vi "user interface.vi"(11 "Serial port assistant view":refnum<class "Serial port assistant view.lvclass">) -> ()   [LabVIEW 2022 SP3, in "Serial port assistant view.lvlib" / "Serial port assistant view.lvclass"]
uses:
  Serial port assistant view.lvclass
  Serial port assistant view.lvclass/Serial port assistant view.ctl
panel:
  in  "open?":bool
  in  "发送间隔":u32
  in  "定时发送？":bool
  in  "HEX？":bool
  in  "清空显示":bool
  in  "HEX显示？":bool
  in  "发送":bool
  in  "发送数据":string
  in  "停止位":string(combo)="1"
  in  "校验位":string(combo)="none"
  in  "数据位":string(combo)="8"
  in  "波特率":string(combo)="9600"
  in  "串口号":string(combo)
  in  "打开串口":bool
  out "实时显示":string
  # "串口设置"
  # "串口设置"
  # "设置"
  # "实时显示"
  # "发送"
  # "发送间隔(ms)"
  # "定时发送"
  # "HEX"
  # "HEX显示"
  # "停止位："
  # "校验位："
  # "数据位："
  # "波特率："
  # "串口号："
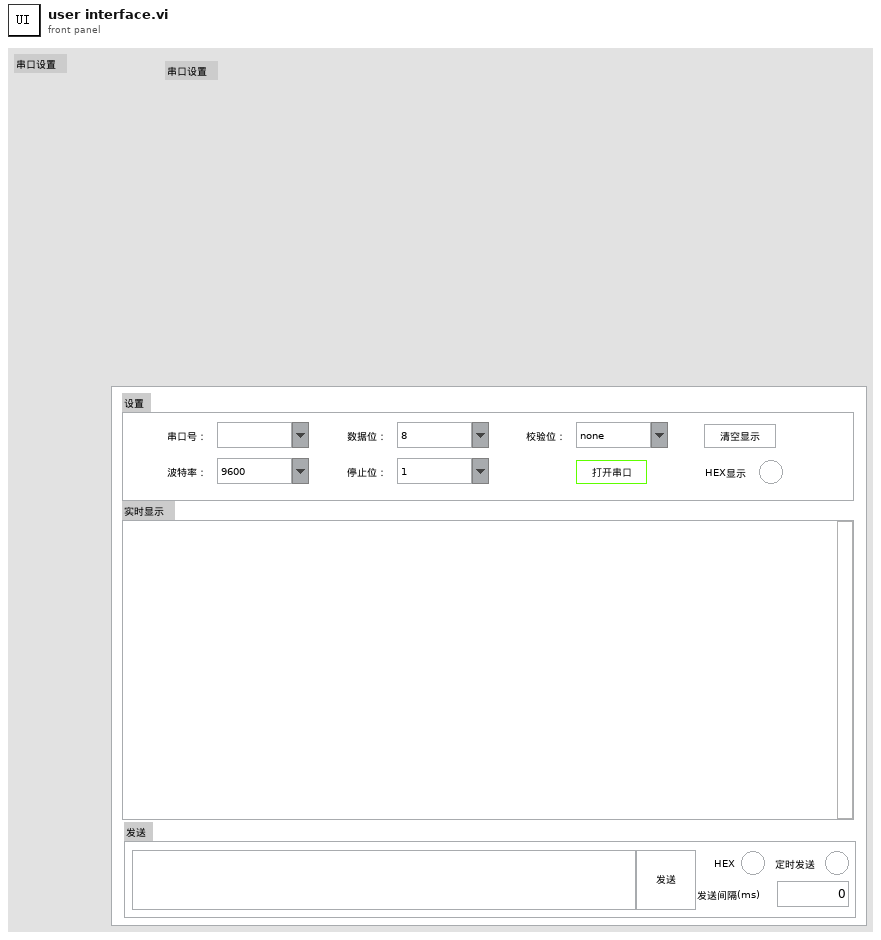
[diagram p1: front panel]
types:
  T1 = cluster{"request":string, "serial port":string, "baud rate":u32, "data bits":u16, "stop bits":u16, "parity":u16}
  T2 = cluster{"request":string, "data to be sent":string}
  T3 = enum8{"Enabled", "Disabled", "Disabled and Grayed Out"}
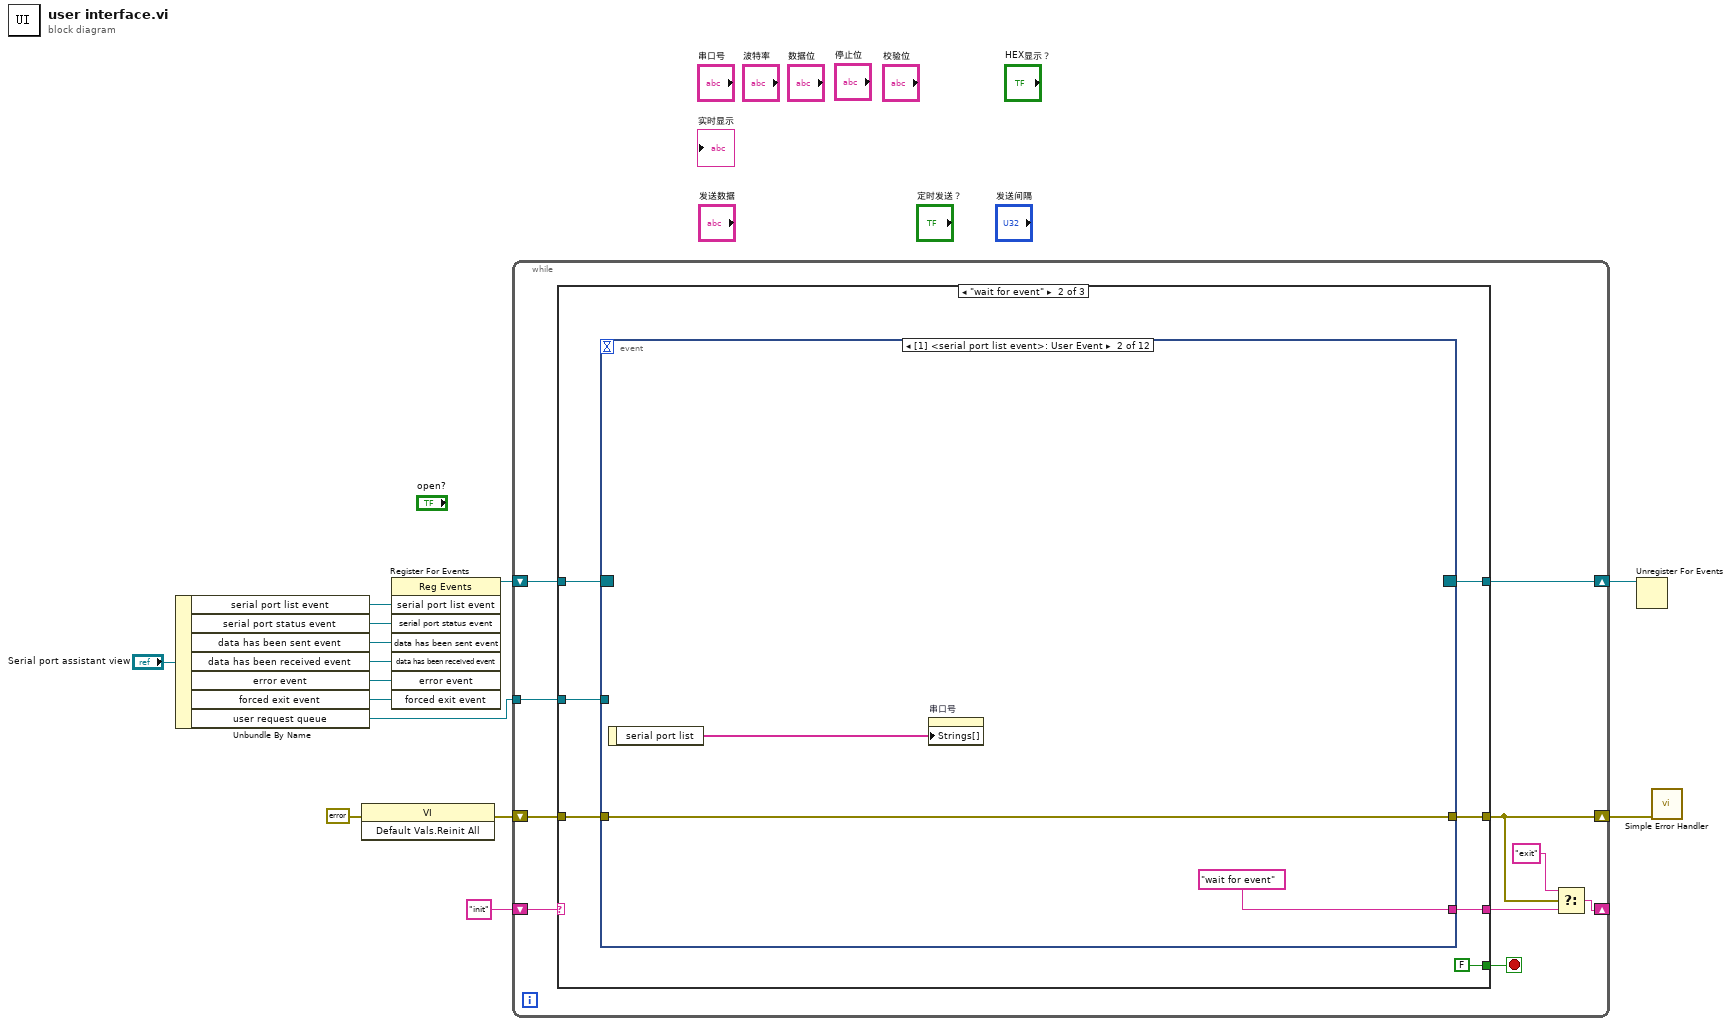
[diagram p0: block diagram]
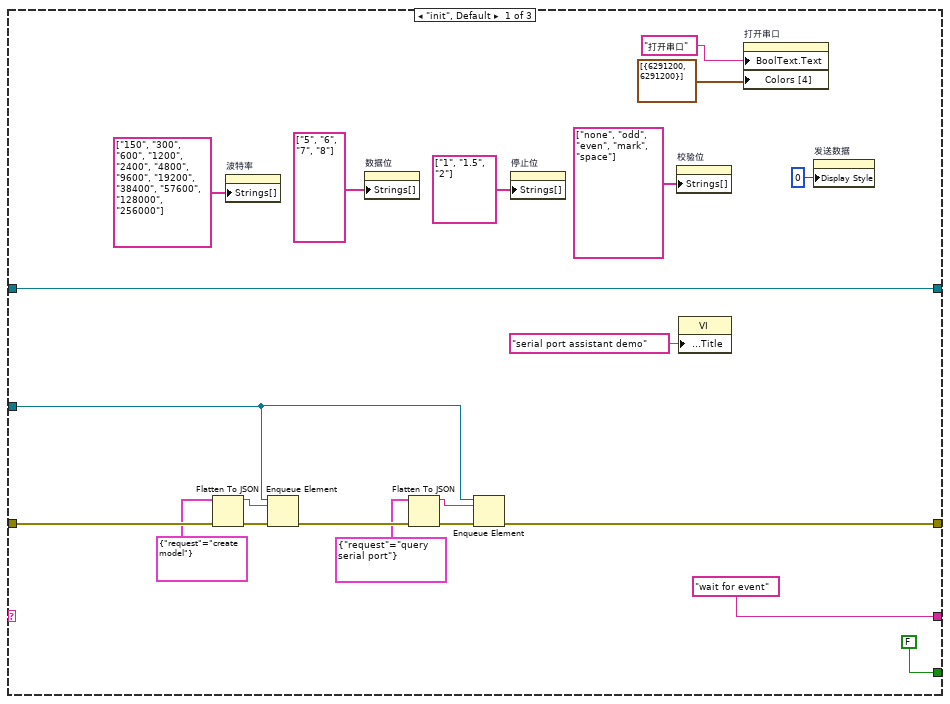
[diagram p2: hidden frame]
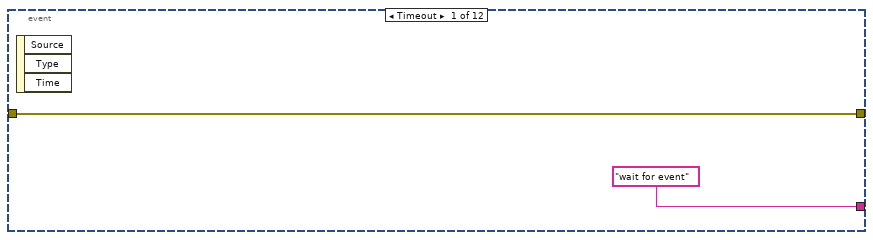
[diagram p3: hidden frame]
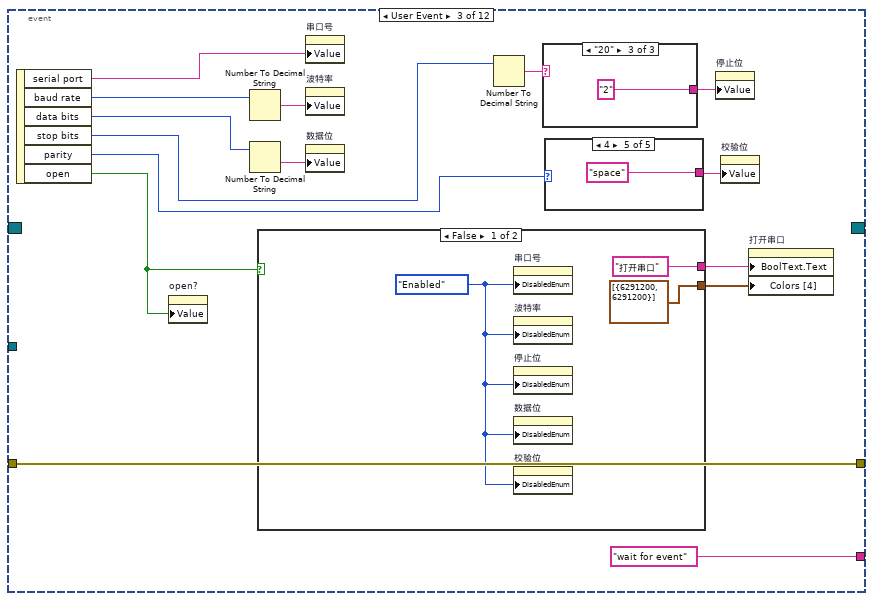
[diagram p4: hidden frame]
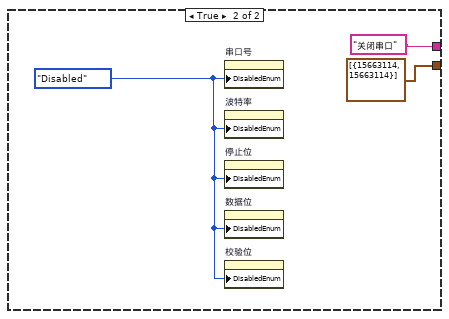
[diagram p5: hidden frame]
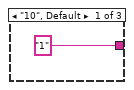
[diagram p6: hidden frame]
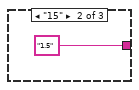
[diagram p7: hidden frame]
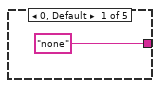
[diagram p8: hidden frame]
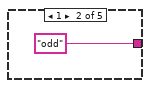
[diagram p9: hidden frame]
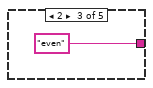
[diagram p10: hidden frame]
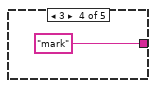
[diagram p11: hidden frame]
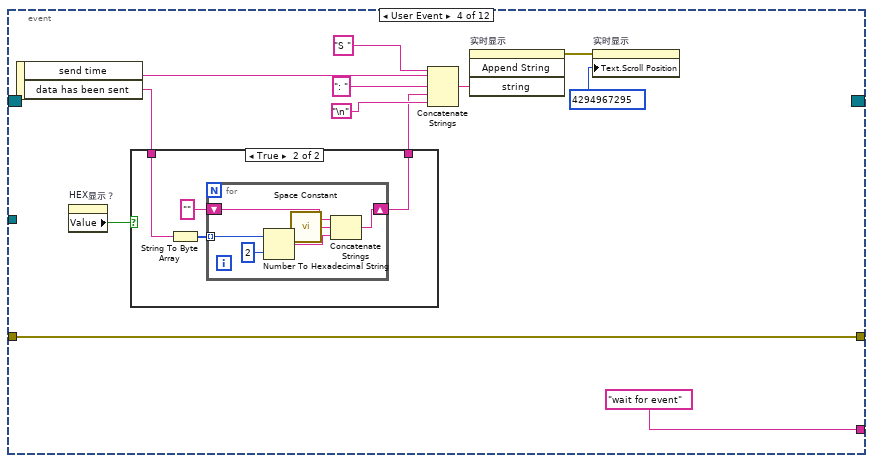
[diagram p12: hidden frame]
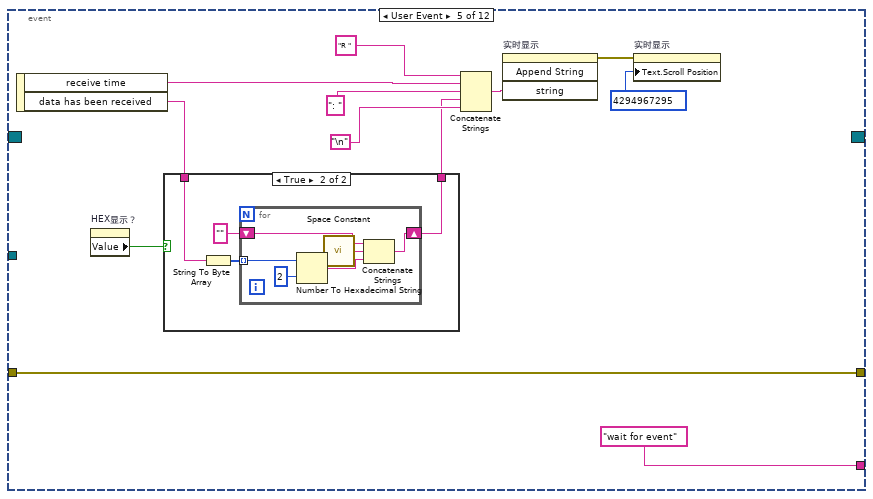
[diagram p14: hidden frame]
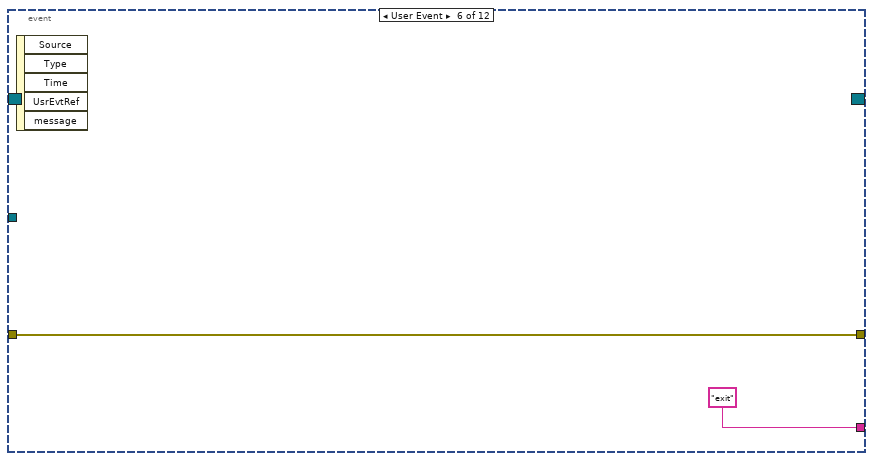
[diagram p16: hidden frame]
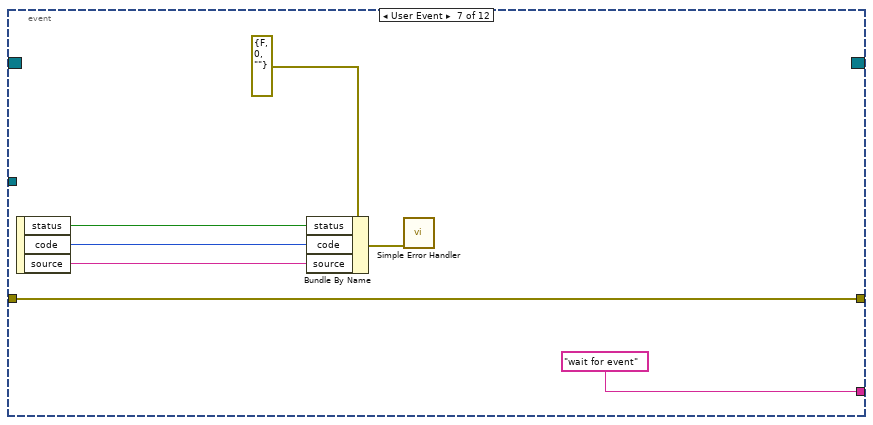
[diagram p17: hidden frame]
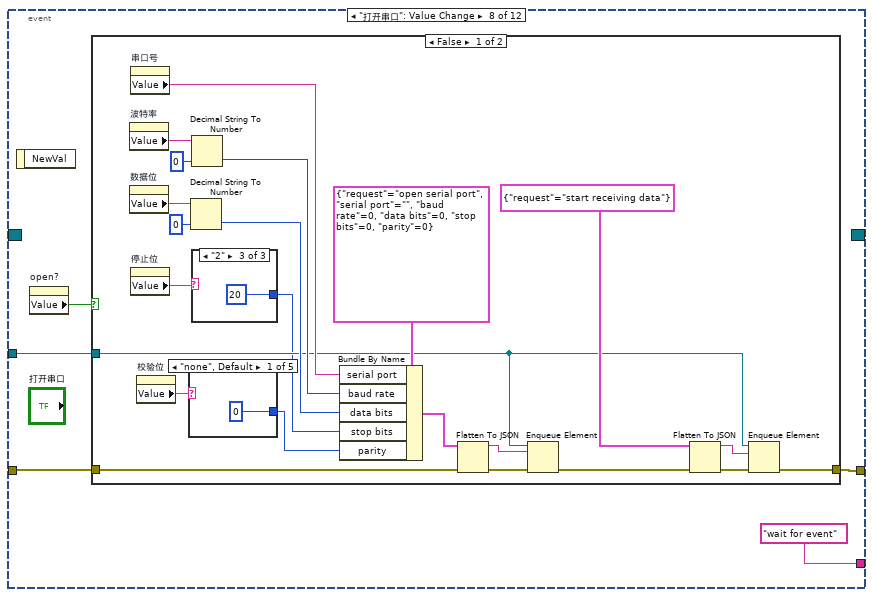
[diagram p18: hidden frame]
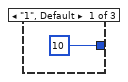
[diagram p19: hidden frame]
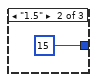
[diagram p20: hidden frame]
diagram:
  n1 = Unbundle By Name("Serial port assistant view") -> ("serial port list event"=w13:refnum<user-event>, "serial port status event"=w12:refnum<user-event>, "data has been sent event"=w11:refnum<user-event>, "data has been received event"=w10:refnum<user-event>, "error event"=w7:refnum<user-event>, "forced exit event"=w2:refnum<user-event>, "user request queue"=w1:refnum<queue>)
  n2 = invoke class="VI" method="Default Vals.Reinit All"(error in=errorcluster {"status"=FALSE, "code"=0, "source"=""} ("error in (no error)")) -> (error out=w5:errorcluster)  [unwired: 2 in, 2 out]
  n3 = register-events(w13, w12, w11, w10, w7, w2) -> (reference out=w9:refnum<event-registration>)  [unwired: 2 in, 1 out]
  n4 = while {
    shift-right: [w19] -> w8
    shift-left: w5 -> [w23]
    tunnel: w1 -> [w22]
    shift-right: [w16] -> _
    shift-left: "init" -> [w21]
    shift-right: [w20] -> w3
    shift-left: w9 -> [w24]
    stop <- w18 stop-if-true
    n5 = case shown="\"wait for event\"" w21 {
      tunnel: w24 -> [w45 w52 w266]
      tunnel: [w45 w51 w266] -> w20
      tunnel: w23 -> [w38 w50 w259]
      tunnel: w22 -> [w37 w49 w261]
      tunnel: [w36 w48 w258] -> w19
      tunnel: [FALSE FALSE TRUE ("Discard?")] -> w18
      tunnel: ["wait for event" w47 "exit"] -> w17
      frame "init", Default {
        n6 = Flatten To JSON(anything=cluster{"request":string} {"request"="create model"}, error in (no error)=w38) -> (JSON string=w43:string, 11:w40:errorcluster)  [unwired: 1 in]
        n7 = property on="波特率" class="CmbBox"("Strings[]"=string[] ["150", "300", "600", "1200", "2400", "4800", "9600", "19200", "38400", "57600", "128000", "256000"] ("Strings [] 5")) -> ()  [unwired: 2 in, 2 out]
        n8 = Enqueue Element(queue=w37, element=w43, error in (no error)=w40) -> (error out=w41:errorcluster)  [unwired: 1 in, 2 out]
        n9 = property on="数据位" class="CmbBox"("Strings[]"=string[] ["5", "6", "7", "8"] ("Strings [] 5")) -> ()  [unwired: 2 in, 2 out]
        n10 = Flatten To JSON(anything=cluster{"request":string} {"request"="query serial port"}, error in (no error)=w41) -> (JSON string=w44:string, 11:w42:errorcluster)  [unwired: 1 in]
        n11 = Enqueue Element(queue=w37, element=w44, error in (no error)=w42) -> (error out=w36:errorcluster)  [unwired: 1 in, 2 out]
        n12 = property on="停止位" class="CmbBox"("Strings[]"=string[] ["1", "1.5", "2"] ("Strings [] 5")) -> ()  [unwired: 2 in, 2 out]
        n13 = property on="校验位" class="CmbBox"("Strings[]"=string[] ["none", "odd", "even", "mark", "space"] ("Strings [] 5")) -> ()  [unwired: 2 in, 2 out]
        n14 = property class="VI"("Front Panel.Title"="serial port assistant demo" ("Front Panel Window:Title")) -> ()  [unwired: 2 in, 2 out]
        n15 = property on="打开串口" class="Bool"("BoolText.Text"="打开串口", "Colors [4]"=cluster{u32, u32}[] [{6291200, 6291200}]) -> ()  [unwired: 2 in, 2 out]
        n16 = property on="发送数据" class="Str"("Display Style"=u32 0) -> ()  [unwired: 2 in, 2 out]
      }
      frame "wait for event" {
        n17 = event shown="[1] <serial port list event>: User Event" {
          selector: w52 -> [_ _ _ _ _ _ _ _ _ _ _ _]
          dyn-events: [_ _ _ _ _ _ _ _ _ _ _ _] -> w51
          timeout: _ -> [_ _ _ _ _ _ _ _ _ _ _ _]
          tunnel: w50 -> [w54 w56 w67 w96 w119 w133 w141 w145 w188 w195 w215 w222]
          tunnel: [w54 w56 w67 w96 w119 w133 w141 w144 w188 w194 w215 w224] -> w48
          tunnel: w49 -> [_ _ _ _ _ _ _ w143 _ w193 _ w223]
          tunnel: ["wait for event" "wait for event" "wait for event" "wait for event" "wait for event" "exit" "wait for event" "wait for event" "wait for event" "wait for event" "wait for event" w220] -> w47
          event Timeout {
            n18 = event-data() -> ()  [unwired: 1 in, 3 out]
          }
          event User Event {
            n19 = event-data() -> ("serial port list"=w57:string[])  [unwired: 1 in]
            n20 = property on="串口号" class="CmbBox"("Strings[]"=w57) -> ()  [unwired: 2 in, 2 out]
          }
          event User Event {
            n21 = event-data() -> ("serial port"=w72:string, "baud rate"=w71:u32, "data bits"=w68:u16, "stop bits"=w58:u16, "parity"=w65:u16, "open"=w61:bool)  [unwired: 1 in]
            n22 = property on="open?" class="Bool (strict)"("Value"=w61) -> ()  [unwired: 2 in, 2 out]
            n23 = Number To Decimal String(number=w71) -> (decimal integer string=w70:string)  [unwired: 1 in]
            n24 = Number To Decimal String(number=w68) -> (decimal integer string=w69:string)  [unwired: 1 in]
            n25 = case shown="False" w61 {
              tunnel: ["打开串口" "关闭串口"] -> w60
              tunnel: [cluster{u32, u32}[] [{6291200, 6291200}] ("Colors [4]") cluster{u32, u32}[] [{15663114, 15663114}] ("Colors [4]")] -> w59
              frame False {
                w73 = T3."Enabled" ("Disabled")
                n26 = property on="串口号" class="CmbBox"("DisabledEnum"=w73) -> ()  [unwired: 2 in, 2 out]
                n27 = property on="波特率" class="CmbBox"("DisabledEnum"=w73) -> ()  [unwired: 2 in, 2 out]
                n28 = property on="停止位" class="CmbBox"("DisabledEnum"=w73) -> ()  [unwired: 2 in, 2 out]
                n29 = property on="数据位" class="CmbBox"("DisabledEnum"=w73) -> ()  [unwired: 2 in, 2 out]
                n30 = property on="校验位" class="CmbBox"("DisabledEnum"=w73) -> ()  [unwired: 2 in, 2 out]
              }
              frame True {
                w76 = T3."Disabled" ("Disabled")
                n31 = property on="串口号" class="CmbBox"("DisabledEnum"=w76) -> ()  [unwired: 2 in, 2 out]
                n32 = property on="波特率" class="CmbBox"("DisabledEnum"=w76) -> ()  [unwired: 2 in, 2 out]
                n33 = property on="停止位" class="CmbBox"("DisabledEnum"=w76) -> ()  [unwired: 2 in, 2 out]
                n34 = property on="数据位" class="CmbBox"("DisabledEnum"=w76) -> ()  [unwired: 2 in, 2 out]
                n35 = property on="校验位" class="CmbBox"("DisabledEnum"=w76) -> ()  [unwired: 2 in, 2 out]
              }
            }
            n36 = property on="串口号" class="CmbBox"("Value"=w72) -> ()  [unwired: 2 in, 2 out]
            n37 = property on="波特率" class="CmbBox"("Value"=w70) -> ()  [unwired: 2 in, 2 out]
            n38 = property on="数据位" class="CmbBox"("Value"=w69) -> ()  [unwired: 2 in, 2 out]
            n39 = Number To Decimal String(number=w58) -> (decimal integer string=w63:string)  [unwired: 1 in]
            n40 = case shown="\"20\"" w63 {
              tunnel: ["1" "1.5" "2"] -> w62
              frame "10", Default {
              }
              frame "15" {
              }
              frame "20" {
              }
            }
            n41 = case shown="4" w65 {
              tunnel: ["none" "odd" "even" "mark" "space"] -> w64
              frame 0, Default {
              }
              frame 1 {
              }
              frame 2 {
              }
              frame 3 {
              }
              frame 4 {
              }
            }
            n42 = property on="停止位" class="CmbBox"("Value"=w62) -> ()  [unwired: 2 in, 2 out]
            n43 = property on="校验位" class="CmbBox"("Value"=w64) -> ()  [unwired: 2 in, 2 out]
            n44 = property on="打开串口" class="Bool"("BoolText.Text"=w60, "Colors [4]"=w59) -> ()  [unwired: 2 in, 2 out]
          }
          event User Event {
            n45 = event-data() -> ("send time"=w92:string, "data has been sent"=w88:string)  [unwired: 1 in]
            n46 = property on="HEX显示？" class="Bool (strict)"() -> ("Value"=w89:bool)  [unwired: 2 in, 2 out]
            n47 = case shown="True" w89 {
              tunnel: w88 -> [w99 w101]
              tunnel: [w99 w100] -> w87
              frame False {
              }
              frame True {
                n48 = String To Byte Array(string=w101) -> (unsigned byte array=w102:u8[])
                n49 = for {
                  tunnel: w102 -> [w108] mode=indexing
                  shift-right: [w106] -> w100
                  shift-left: "" -> [w107]
                  n50 = Number To Hexadecimal String(1:i16 2 ("width (-)"), 2:w108) -> (0:w105:string)
                  n51 = call <vilib>:"Space Constant.vi"() -> ("String"=w104:string)
                  n52 = Concatenate Strings(w107, w104, w105) -> (w106:string)
                }
              }
            }
            n53 = Concatenate Strings("S " ("string"), w92, ": ", w87, "\n") -> (w94:string)
            n54 = invoke on="实时显示" class="Str" method="Append String"("string"=w94) -> (error out=w98:errorcluster)  [unwired: 3 in, 3 out]
            n55 = property on="实时显示" class="Str"(error in=w98, "Text.Scroll Position"=u32 4294967295) -> ()  [unwired: 1 in, 2 out]
          }
          event User Event {
            n56 = event-data() -> ("receive time"=w114:string, "data has been received"=w111:string)  [unwired: 1 in]
            n57 = property on="HEX显示？" class="Bool (strict)"() -> ("Value"=w112:bool)  [unwired: 2 in, 2 out]
            n58 = case shown="True" w112 {
              tunnel: w111 -> [w122 w124]
              tunnel: [w122 w123] -> w110
              frame False {
              }
              frame True {
                n59 = String To Byte Array(string=w124) -> (unsigned byte array=w125:u8[])
                n60 = for {
                  tunnel: w125 -> [w131] mode=indexing
                  shift-right: [w129] -> w123
                  shift-left: "" -> [w130]
                  n61 = Number To Hexadecimal String(1:i16 2 ("width (-)"), 2:w131) -> (0:w128:string)
                  n62 = call <vilib>:"Space Constant.vi"() -> ("String"=w127:string)
                  n63 = Concatenate Strings(w130, w127, w128) -> (w129:string)
                }
              }
            }
            n64 = Concatenate Strings("R " ("string"), w114, ": ", w110, "\n") -> (w113:string)
            n65 = invoke on="实时显示" class="Str" method="Append String"("string"=w113) -> (error out=w121:errorcluster)  [unwired: 3 in, 3 out]
            n66 = property on="实时显示" class="Str"(error in=w121, "Text.Scroll Position"=u32 4294967295) -> ()  [unwired: 1 in, 2 out]
          }
          event User Event {
            n67 = event-data() -> ()  [unwired: 1 in, 5 out]
          }
          event User Event {
            n68 = event-data() -> ("status"=w139:bool, "code"=w138:i32, "source"=w137:string)  [unwired: 1 in]
            n69 = Bundle By Name(cluster=errorcluster {"status"=FALSE, "code"=0, "source"=""} ("error in (no error)"), "status"=w139, "code"=w138, "source"=w137) -> (w136:errorcluster)
            n70 = call <vilib>:"Simple Error Handler.vi"("error in (no error)"=w136) -> ()  [unwired: 4 in, 5 out]
          }
          event "打开串口": Value Change {
            n71 = event-data() -> ()  [unwired: 1 in, 1 out]
            n72 = property on="open?" class="Bool (strict)"() -> ("Value"=w142:bool)  [unwired: 2 in, 2 out]
            n73 = case shown="False" w142 {
              tunnel: w145 -> [w166 w184]
              tunnel: [w153 w180] -> w144
              tunnel: w143 -> [w154 w177]
              frame False {
                n74 = property on="波特率" class="CmbBox"() -> ("Value"=w164:string)  [unwired: 2 in, 2 out]
                n75 = property on="数据位" class="CmbBox"() -> ("Value"=w162:string)  [unwired: 2 in, 2 out]
                n76 = property on="串口号" class="CmbBox"() -> ("Value"=w165:string)  [unwired: 2 in, 2 out]
                n77 = property on="停止位" class="CmbBox"() -> ("Value"=w148:string)  [unwired: 2 in, 2 out]
                n78 = property on="校验位" class="CmbBox"() -> ("Value"=w150:string)  [unwired: 2 in, 2 out]
                n79 = case shown="\"none\", Default" w150 {
                  tunnel: [u16 0 u16 1 u16 2 u16 3 u16 4] -> w149
                  frame "none", Default {
                  }
                  frame "odd" {
                  }
                  frame "even" {
                  }
                  frame "mark" {
                  }
                  frame "space" {
                  }
                }
                n80 = Decimal String To Number(string=w162, default (0L)=u16 0 ("default (0 I32)")) -> (number=w161:u16)  [unwired: 1 in, 1 out]
                n81 = Decimal String To Number(string=w164, default (0L)=u32 0 ("default (0 I32)")) -> (number=w163:u32)  [unwired: 1 in, 1 out]
                n82 = case shown="\"2\"" w148 {
                  tunnel: [u16 10 ("default (0 I32)") u16 15 ("default (0 I32)") u16 20 ("default (0 I32)")] -> w147
                  frame "1", Default {
                  }
                  frame "1.5" {
                  }
                  frame "2" {
                  }
                }
                n83 = Bundle By Name(cluster=T1 {"request"="open serial port", "serial port"="", "baud rate"=0, "data bits"=0, "stop bits"=0, "parity"=0}, "serial port"=w165, "baud rate"=w163, "data bits"=w161, "stop bits"=w147, "parity"=w149) -> (w160:T1)
                n84 = Flatten To JSON(anything=w160, error in (no error)=w166) -> (JSON string=w168:string, 11:w167:errorcluster)  [unwired: 1 in]
                n85 = Enqueue Element(queue=w154, element=w168, error in (no error)=w167) -> (error out=w158:errorcluster)  [unwired: 1 in, 2 out]
                n86 = Flatten To JSON(anything=cluster{"request":string} {"request"="start receiving data"}, error in (no error)=w158) -> (JSON string=w156:string, 11:w157:errorcluster)  [unwired: 1 in]
                n87 = Enqueue Element(queue=w154, element=w156, error in (no error)=w157) -> (error out=w153:errorcluster)  [unwired: 1 in, 2 out]
              }
              frame True {
                n88 = Flatten To JSON(anything=cluster{"request":string} {"request"="stop receiving data"}, error in (no error)=w184) -> (JSON string=w185:string, 11:w186:errorcluster)  [unwired: 1 in]
                n89 = Enqueue Element(queue=w177, element=w185, error in (no error)=w186) -> (error out=w181:errorcluster)  [unwired: 1 in, 2 out]
                n90 = Flatten To JSON(anything=cluster{"request":string} {"request"="close serial port"}, error in (no error)=w181) -> (JSON string=w182:string, 11:w179:errorcluster)  [unwired: 1 in]
                n91 = Enqueue Element(queue=w177, element=w182, error in (no error)=w179) -> (error out=w180:errorcluster)  [unwired: 1 in, 2 out]
              }
            }
          }
          event "清空显示": Value Change {
            n92 = event-data() -> ()  [unwired: 1 in, 1 out]
            n93 = property on="实时显示" class="Str"("Value"="") -> ()  [unwired: 2 in, 2 out]
          }
          event "发送": Value Change {
            n94 = event-data() -> ()  [unwired: 1 in, 1 out]
            n95 = property on="open?" class="Bool (strict)"() -> ("Value"=w190:bool)  [unwired: 2 in, 2 out]
            n96 = And(x="发送", y=w190) -> (x .and. y?=w191:bool)
            n97 = case shown="True" w191 {
              tunnel: w195 -> [w199 w201]
              tunnel: [w199 w202] -> w194
              tunnel: w193 -> [_ w203]
              frame False {
                n98 = One Button Dialog(message="请先打开串口", button name ("OK")="继续") -> ()  [unwired: 1 out]
              }
              frame True {
                n99 = property on="发送数据" class="Str"() -> ("Value"=w200:string)  [unwired: 2 in, 2 out]
                n100 = case shown="\"other\", Default" w200 {
                  selector: w200 -> [_ w207]
                  tunnel: w203 -> [_ w210]
                  tunnel: [w206 w209] -> w202
                  tunnel: w201 -> [w206 w208]
                  frame "" {
                    n101 = One Button Dialog(message="待发送数据为空！", button name ("OK")="继续") -> ()  [unwired: 1 out]
                  }
                  frame "other", Default {
                    n102 = Bundle By Name(cluster=T2 {"request"="send data", "data to be sent"=""}, "data to be sent"=w207) -> (w211:T2)
                    n103 = Flatten To JSON(anything=w211, error in (no error)=w208) -> (JSON string=w213:string, 11:w214:errorcluster)  [unwired: 1 in]
                    n104 = Enqueue Element(queue=w210, element=w213, error in (no error)=w214) -> (error out=w209:errorcluster)  [unwired: 1 in, 2 out]
                  }
                }
              }
            }
          }
          event "HEX？": Value Change {
            n105 = event-data() -> ()  [unwired: 1 in, 6 out]
            n106 = case shown="False" "HEX？" {
              frame False {
                n107 = property on="发送数据" class="Str"("Display Style"=u32 0) -> ()  [unwired: 2 in, 2 out]
              }
              frame True {
                n108 = property on="发送数据" class="Str"("Display Style"=u32 3) -> ()  [unwired: 2 in, 2 out]
              }
            }
          }
          event Panel Close? {
            n109 = event-data() -> ()  [unwired: 1 in, 1 out]
            n110 = property on="open?" class="Bool (strict)"() -> ("Value"=w221:bool)  [unwired: 2 in, 2 out]
            n111 = case shown="True" w221 {
              tunnel: [w232 w234] -> w224
              tunnel: w223 -> [w231 w235]
              tunnel: w222 -> [w230 w236]
              tunnel: ["exit" w233] -> w220
              frame False {
                n112 = Flatten To JSON(anything=cluster{"request":string} {"request"="destroy model"}, error in (no error)=w230) -> (JSON string=w227:string, 11:w229:errorcluster)  [unwired: 1 in]
                n113 = Enqueue Element(queue=w231, element=w227, error in (no error)=w229) -> (error out=w232:errorcluster)  [unwired: 1 in, 2 out]
              }
              frame True {
                n114 = Two Button Dialog(message="串口正在使用中，是否关闭程序？", 1:"否" ("F button name (\"Cancel\")"), 2:"是" ("T button name (\"OK\")")) -> (T button?=w237:bool)
                n115 = case shown="True" w237 {
                  tunnel: w236 -> [w242 w248]
                  tunnel: w235 -> [_ w246]
                  tunnel: [w242 w254] -> w234
                  tunnel: ["wait for event" "exit"] -> w233
                  frame False {
                  }
                  frame True {
                    n116 = Flatten To JSON(anything=cluster{"request":string} {"request"="stop receiving data"}, error in (no error)=w248) -> (JSON string=w245:string, 11:w249:errorcluster)  [unwired: 1 in]
                    n117 = Enqueue Element(queue=w246, element=w245, error in (no error)=w249) -> (error out=w247:errorcluster)  [unwired: 1 in, 2 out]
                    n118 = Flatten To JSON(anything=cluster{"request":string} {"request"="close serial port"}, error in (no error)=w247) -> (JSON string=w252:string, 11:w253:errorcluster)  [unwired: 1 in]
                    n119 = Enqueue Element(queue=w246, element=w252, error in (no error)=w253) -> (error out=w251:errorcluster)  [unwired: 1 in, 2 out]
                    n120 = Flatten To JSON(anything=cluster{"request":string} {"request"="destroy model"}, error in (no error)=w251) -> (JSON string=w255:string, 11:w257:errorcluster)  [unwired: 1 in]
                    n121 = Enqueue Element(queue=w246, element=w255, error in (no error)=w257) -> (error out=w254:errorcluster)  [unwired: 1 in, 2 out]
                  }
                }
              }
            }
            n122 = event-data("Discard?"=TRUE) -> ()  [unwired: 1 in, 1 out]
          }
        }
      }
      frame "exit" {
        n123 = Flatten To JSON(anything=cluster{"request":string} {"request"="exit"}) -> (JSON string=w262:string)  [unwired: 2 in, 1 out]
        n124 = Enqueue Element(queue=w261, element=w262) -> (error out=w260:errorcluster)  [unwired: 2 in, 2 out]
        n125 = Merge Errors(w260, w259) -> (w258:errorcluster)
      }
    }
    n126 = Select(t="exit", s=w19, f=w17) -> (s? t:f=w16:string)
  }
  n127 = Unregister For Events(event registration refnum=w3) -> ()  [unwired: 1 in, 1 out]
  n128 = call <vilib>:"Simple Error Handler.vi"("error in (no error)"=w8) -> ()  [unwired: 4 in, 5 out]
